vi "3DPredictedClassification.vi"(8 "error in":errorcluster, 11 "Parameters":T2={"Parameter"={"3D Plot"=[], "3D Scatter"=refnum, "Data"={"X"=[], "Predict"=[]}, "Display"={"Choice"=enum."All", "Indexe"={"X"=0, "Y"=1, "Z"=2}}, "Point Property"={"Style"=enum."Full circle", "Label Color"=[8978528, 4367871, 1985280]}}}) -> (0 "error out":errorcluster, 3 "Local Out":T2={"Parameter"={"3D Plot"=[], "3D Scatter"=refnum, "Data"={"X"=[], "Predict"=[]}, "Display"={"Choice"=enum."All", "Indexe"={"X"=0, "Y"=0, "Z"=0}}, "Point Property"={"Style"=enum."Full circle", "Label Color"=[8978528, 4367871, 1985280]}}})   [LabVIEW 2020]
doc: "Displays the predicted data in 3D"
uses:
  <vilib>/Math Plots/3D Math Plots/3D Plot/3D Plot Datatype/3D Plot Datatype.lvclass
  <vilib>/Math Plots/3D Math Plots/3D Scatter/3D Scatter XCtrl/3D Scatter.xctl
  _Controls/Style.ctl
  <vilib>/Math Plots/3D Math Plots/3D Plot/3D Plot/Typedef/Color Ramp Cluster.ctl
  <vilib>/Math Plots/3D Math Plots/3D Plot/3D Plot/3D Plot.lvclass
types:
  T1 = typedef "Style.ctl" = enum16{"Empty circle", "Full circle", "Empty square", "Full square", "Cross"}
  T2 = cluster{"Parameter":cluster{"3D Plot":refnum<class "3D Plot Datatype.lvclass">[], "3D Scatter":refnum<vi>, "Data":cluster{"X":dbl[][], "Predict":dbl[][]}, "Display":cluster{"Choice":enum16{"All", "Train", "Test"}, "Indexe":cluster{"X":i32, "Y":i32, "Z":i32}}, "Point Property":cluster{"Style":T1, "Label Color":u32[]}}}
  T3 = typedef "3D Plot.lvclass/Color Ramp Cluster.ctl" = cluster{"Color Ramp Style":enum16{"None", "Shaded", "Color spectrum", "Grey scale", "Custom"}, "Color Ramp Array":u32[], "Color Ramp Index":i32[], "Interpolate?":bool, "Logarithm?":bool}
  T4 = typedef "3D Plot.lvclass/Sprite Type.ctl" = enum16{"None", "Empty Square", "Solid Square", "Empty Diamond", "Solid Diamond", "Empty Circle", "Solid Circle", "Asterisk", "Bold X", "Wireframe Sphere", "Solid Sphere", "Wireframe Cube", "Solid Cube"}
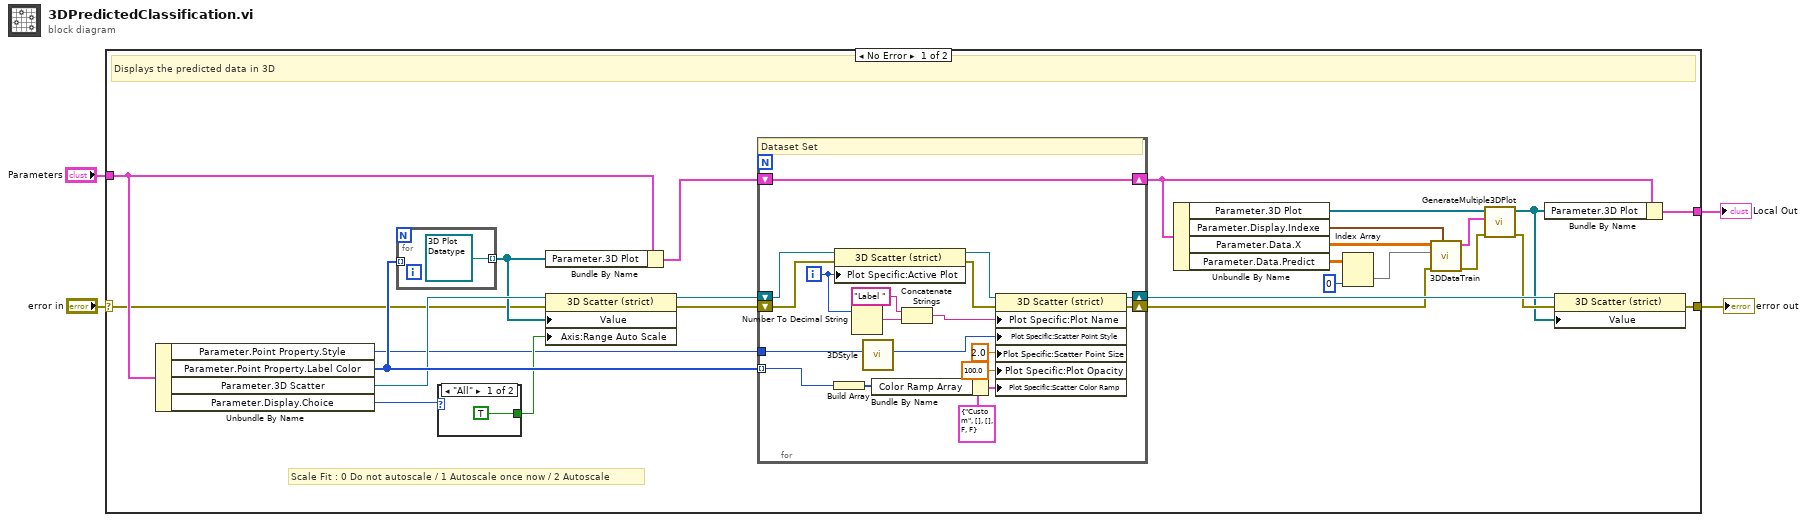
[diagram p0: block diagram]
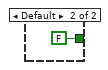
[diagram p2: hidden frame]
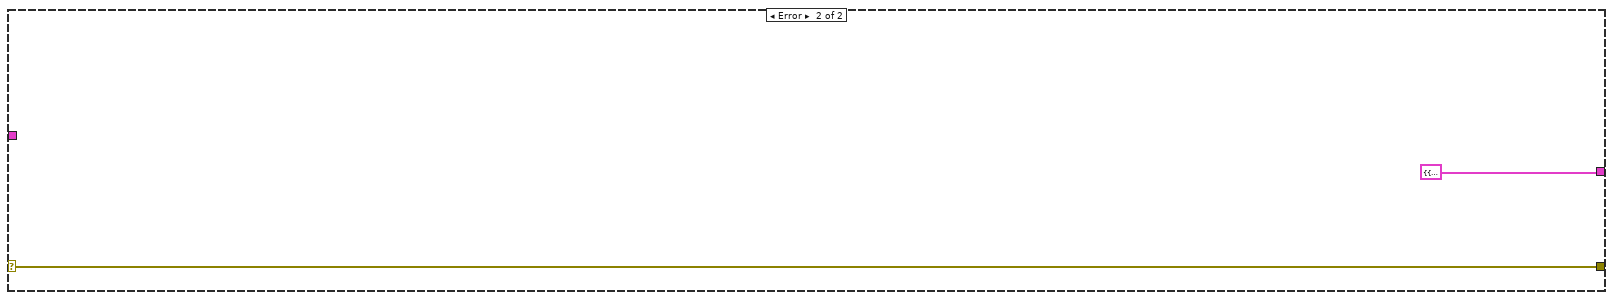
[diagram p3: hidden frame]
diagram:
  n1 = case shown="No Error" "error in" {
    selector: "error in" -> [w16 w54]
    tunnel: [w7 w54] -> w3
    tunnel: "Parameters" -> [w17 _]
    tunnel: [w5 T2 {"Parameter"={"3D Plot"=[], "3D Scatter"=refnum, "Data"={"X"=[], "Predict"=[]}, "Display"={"Choice"=enum."All", "Indexe"={"X"=0, "Y"=0, "Z"=0}}, "Point Property"={"Style"=enum."Empty circle", "Label Color"=[]}}} ("Parameters")] -> w1
    frame No Error {
      # "Scale Fit : 0 Do not autoscale / 1 Autoscale once now / 2 Autoscale"
      # "Displays the predicted data in 3D"
      n2 = Unbundle By Name(w17) -> ("Parameter.Point Property.Style"=w6:T1, "Parameter.Point Property.Label Color"=w30:u32[], "Parameter.3D Scatter"=w20:refnum<vi>, "Parameter.Display.Choice"=w29:enum16{"All", "Train", "Test"})
      n3 = for {
        tunnel: [refnum<class "3D Plot Datatype.lvclass"> refnum ("3D Plot Datatype.lvclass")] -> w19 mode=indexing
        tunnel: w30 -> [_] mode=indexing
      }
      n4 = case shown="\"All\"" w29 {
        tunnel: [TRUE ("x = y?") FALSE ("x = y?")] -> w18
        frame "All" {
        }
        frame Default {
        }
      }
      n5 = Bundle By Name(cluster=w17, "Parameter.3D Plot"=w19) -> (w27:T2)
      n6 = property class="3D Scatter (strict)"(reference=w20, error in=w16, "Value"=w19, "Axis:Range Auto Scale"=w18) -> (reference out=w28:refnum<vi>, error out=w25:errorcluster)
      n7 = for {
        tunnel: w30 -> [w38] mode=indexing
        shift-right: [w49] -> w26
        shift-left: w27 -> [w49]
        shift-right: [w47] -> w24
        shift-left: w28 -> [w46]
        shift-right: [w50] -> w9
        shift-left: w25 -> [w39]
        tunnel: w6 -> [w37]
        i -> [w34]
        # "Dataset Set"
        n8 = Build Array(w38) -> (w43:u32[])
        n9 = property class="3D Scatter (strict)"(reference=w46, error in=w39, "Plot Specific:Active Plot"=w34) -> (reference out=w45:refnum<vi>, error out=w44:errorcluster)
        n10 = Number To Decimal String(number=w34) -> (decimal integer string=w33:string)  [unwired: 1 in]
        n11 = call "3DStyle.vi"("Style"=w37) -> ("Scatter Point Style"=w36:T4)  [unwired: 10 in]
        n12 = Bundle By Name(cluster=T3 {"Color Ramp Style"=enum."Custom", "Color Ramp Array"=[], "Color Ramp Index"=[], "Interpolate?"=FALSE, "Logarithm?"=FALSE} ("Spécifique à un tracé:Nuage:Rampe de couleur du nuage"), "Color Ramp Array"=w43) -> (w41:T3)
        n13 = Concatenate Strings("Label " ("string"), w33) -> (w32:string)
        n14 = property class="3D Scatter (strict)"(reference=w45, error in=w44, "Plot Specific:Plot Name"=w32, "Plot Specific:Scatter Point Style"=w36, "Plot Specific:Scatter Point Size"=sgl 2.0 ("Plot Specific:Scatter:Scatter Point Size"), "Plot Specific:Plot Opacity"=sgl 100.0 ("Plot Specific:General:Plot Opacity"), "Plot Specific:Scatter Color Ramp"=w41) -> (reference out=w47:refnum<vi>, error out=w50:errorcluster)
      }
      n15 = Unbundle By Name(w26) -> ("Parameter.3D Plot"=w23:refnum<class "3D Plot Datatype.lvclass">[], "Parameter.Display.Indexe"=w13:cluster{"X":i32, "Y":i32, "Z":i32}, "Parameter.Data.X"=w12:dbl[][], "Parameter.Data.Predict"=w11:dbl[][])
      n16 = Index Array(array=w11, index (col)=0 ("disabled index (col)")) -> (element=w14:dbl[])  [unwired: 1 in]
      n17 = call "3DDataTrain.vi"("Index"=w13, "error in"=w9, "Y"=w14, "X"=w12) -> ("error out"=w8:errorcluster, "3DArray"=w10:cluster{"X":dbl[], "Y":dbl[], "Z":dbl[]}[])  [unwired: 6 in]
      n18 = call "GenerateMultiple3DPlot.vi"("error in"=w8, "3D Array"=w10, "3D Scatter"=w23) -> ("error out"=w22:errorcluster, "3D Scatter Out"=w21:refnum<class "3D Plot Datatype.lvclass">[])  [unwired: 7 in]
      n19 = Bundle By Name(cluster=w26, "Parameter.3D Plot"=w21) -> (w5:T2)
      n20 = property class="3D Scatter (strict)"(reference=w24, error in=w22, "Value"=w21) -> (error out=w7:errorcluster)  [unwired: 1 out]
    }
    frame Error {
    }
  }
  "error out" <- w3
  "Local Out" <- w1
